vi "Calling Class Methods.vi"() -> ()   [LabVIEW 2020]
uses:
  6d5f1638-640c-4e20-b011-0cee3ae60b95.vi
  688a6956-cd2d-4b8a-a8be-e172edc5432f.vi
  2e819b81-fe13-4050-befc-599fc726c07c.vi
  G-Embedded-Python-Interpreter-Toolkit/Null Py Object Refnum.vi
  6d5f1638-640c-4e20-b011-0cee3ae60b95.vi/96ddca92-7bbf-40e2-a1a5-d32f291eb6af.vi
  688a6956-cd2d-4b8a-a8be-e172edc5432f.vi/6c7a13f1-33d3-431d-8188-904cac5422b3.vi
  G-Embedded-Python-Interpreter-Toolkit/Python Object Reference to Pointer Sized Ref.vi
  2e819b81-fe13-4050-befc-599fc726c07c.vi/6c7a13f1-33d3-431d-8188-904cac5422b3.vi
  G-Embedded-Python-Interpreter-Toolkit/Pointer Sized Ref to Python Object Reference.vi
  G-Embedded-Python-Interpreter-Toolkit/Merge Call Library Errors.vi
  G-Embedded-Python-Interpreter-Toolkit/Generate Argument Type Info.vi
  G-Embedded-Python-Interpreter-Toolkit/G-Embedded-Python-Interpreter-Toolkit.lvlib
panel:
  in  "Decrement":bool
  in  "Increment":bool
  out "Counter Value":i32 format="%011d"
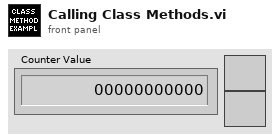
[diagram p1: front panel]
types:
  T1 = typedef "G-Embedded-Python-Interpreter-Toolkit.lvlib/Python Object Reference.ctl" = refnum<k1>
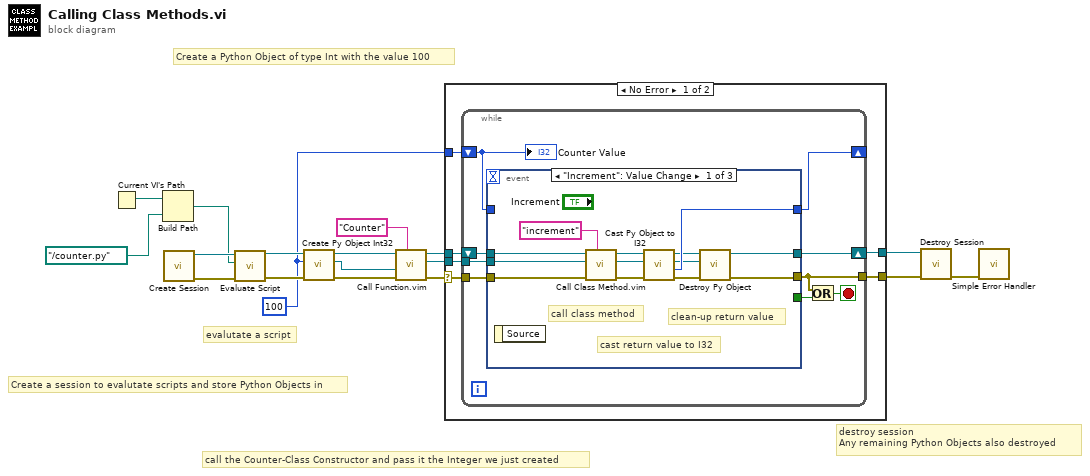
[diagram p0: block diagram]
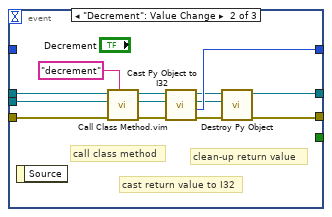
[diagram p2: hidden frame]
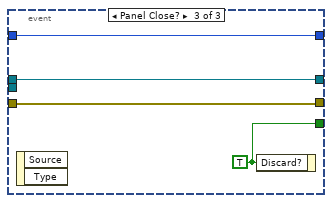
[diagram p3: hidden frame]
diagram:
  w8 = 100 ("Value")
  # "destroy session \nAny remaining Python Objects also destroyed"
  # "Create a Python Object of type Int with the value 100"
  # "call the Counter-Class Constructor and pass it the Integer we just created"
  # "evalutate a script"
  # "Create a session to evalutate scripts and store Python Objects in"
  n1 = Current VI's Path() -> (path=w16:path)
  n2 = Build Path(base path=w16, name or relative path=path "../counter.py") -> (appended path=w14:path)
  n3 = call "Create Session.vi"() -> ("error out"=w18:errorcluster, "Session Handle"=w17:refnum<data-value>)  [unwired: 10 in]
  n4 = call "Evaluate Script.vi"("error in (no error)"=w18, "Script File Path"=w14, "Session Handle in"=w17) -> ("error out"=w11:errorcluster, "Session Handle out"=w12:refnum<data-value>)  [unwired: 7 in]
  n5 = call "Create Py Object Int32.vi"("error in (no error)"=w11, "Value"=w8, "Session Handle in"=w12) -> ("error out"=w10:errorcluster, "Python Object Refnum"=w1:T1, "Session Handle out"=w9:refnum<data-value>)  [unwired: 6 in]
  n6 = call "Call Function.vim"("Function Name"="Counter", "error in (no error)"=w10, "Arguments in (Default - None)"=w1, "Data Value Reference in"=w9) -> ("error out"=w7:errorcluster, "Returned Python Object Refnum"=w5:T1, "Data Value Reference out"=w6:refnum<data-value>)  [unwired: 5 in]
  n7 = case shown="No Error" w7 {
    selector: w7 -> [w23 w65]
    tunnel: w8 -> [w24 _]
    tunnel: w6 -> [w22 w64]
    tunnel: w5 -> [w21 _]
    tunnel: [w20 w65] -> w4
    tunnel: [w19 w64] -> w3
    frame No Error {
      n8 = while {
        tunnel: w23 -> [w33]
        shift-right: [w28] -> w19
        shift-left: w22 -> [w32]
        tunnel: w21 -> [w31]
        shift-right: [w30] -> _
        shift-left: w24 -> [w27]
        tunnel: [w25] -> w20
        stop <- w29 stop-if-true
        n9 = event shown="[0] \"Increment\": Value Change" {
          selector: _ -> [_ _ _]
          dyn-events: _ -> [_ _ _]
          timeout: _ -> [_ _ _]
          tunnel: w33 -> [w46 w59 w63]
          tunnel: w32 -> [w45 w58 w62]
          tunnel: w31 -> [w44 w57 _]
          tunnel: [w39 w52 w61] -> w30
          tunnel: [w35 w48 w63] -> w25
          tunnel: [w34 w47 w62] -> w28
          tunnel: w27 -> [_ _ w61]
          tunnel: [_ _ w60] -> w26
          event "Increment": Value Change {
            # "clean-up return value"
            # "cast return value to I32"
            # "call class method"
            n10 = event-data() -> ()  [unwired: 1 in, 1 out]
            n11 = call "Call Class Method.vim"("Function Name"="increment", "error in (no error)"=w46, "Class Instance"=w44, "Data Value Reference in"=w45) -> ("error out"=w42:errorcluster, "Returned Python Object Refnum"=w40:T1, "Data Value Reference out"=w41:refnum<data-value>)  [unwired: 5 in]
            n12 = call "Cast Py Object to I32.vi"("error in (no error)"=w42, "Python Object Refnum in"=w40, "Session Handle in"=w41) -> ("error out"=w36:errorcluster, "Value"=w39:i32, "Python Object Refnum out"=w37:T1, "Session Handle out"=w38:refnum<data-value>)  [unwired: 5 in]
            n13 = call "Destroy Py Object.vi"("error in (no error)"=w36, "Python Object Refnum"=w37, "Session Handle in"=w38) -> ("error out"=w35:errorcluster, "Session Handle out"=w34:refnum<data-value>)  [unwired: 7 in]
          }
          event "Decrement": Value Change {
            # "clean-up return value"
            # "cast return value to I32"
            # "call class method"
            n14 = event-data() -> ()  [unwired: 1 in, 1 out]
            n15 = call "Call Class Method.vim"("Function Name"="decrement", "error in (no error)"=w59, "Class Instance"=w57, "Data Value Reference in"=w58) -> ("error out"=w55:errorcluster, "Returned Python Object Refnum"=w53:T1, "Data Value Reference out"=w54:refnum<data-value>)  [unwired: 5 in]
            n16 = call "Cast Py Object to I32.vi"("error in (no error)"=w55, "Python Object Refnum in"=w53, "Session Handle in"=w54) -> ("error out"=w49:errorcluster, "Value"=w52:i32, "Python Object Refnum out"=w50:T1, "Session Handle out"=w51:refnum<data-value>)  [unwired: 5 in]
            n17 = call "Destroy Py Object.vi"("error in (no error)"=w49, "Python Object Refnum"=w50, "Session Handle in"=w51) -> ("error out"=w48:errorcluster, "Session Handle out"=w47:refnum<data-value>)  [unwired: 7 in]
          }
          event Panel Close? {
            w60 = TRUE ("Discard?")
            n18 = event-data() -> ()  [unwired: 1 in, 2 out]
            n19 = event-data("Discard?"=w60) -> ()  [unwired: 1 in, 1 out]
          }
        }
        n20 = Or(x=w25, y=w26) -> (x .or. y?=w29:bool)
        "Counter Value" <- w27
      }
    }
    frame Error {
    }
  }
  n21 = call "Destroy Session.vi"("error in (no error)"=w4, "Session Handle"=w3) -> ("error out"=w2:errorcluster)  [unwired: 9 in]
  n22 = call <vilib>:"Simple Error Handler.vi"("error in (no error)"=w2) -> ()  [unwired: 4 in, 5 out]
